vi "string to power value.vi"(9 "String":string) -> (10 "Power":T1)   [LabVIEW 2011]
uses:
  Power_config.ctl
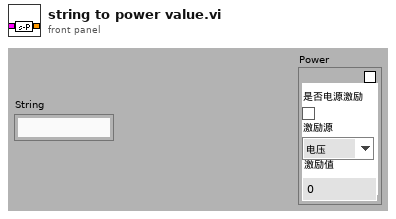
[diagram p1: front panel]
types:
  T1 = typedef "Power_config.ctl" = cluster{"power_en":bool, "Mode":enum16{"电压", "电流"}, "value":dbl, "Boolean":bool}
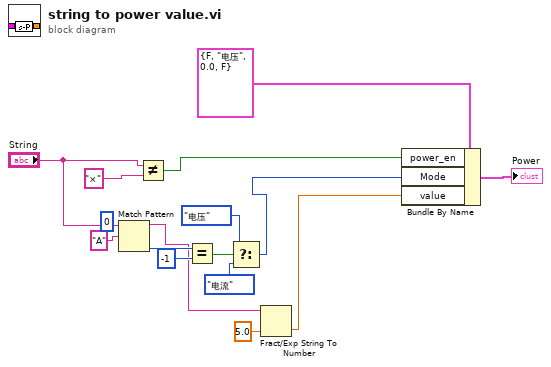
[diagram p0: block diagram]
diagram:
  (unwired) 0 ("offset past match")
  n1 = Match Pattern(string="String", regular expression="A") -> (before substring=w3:string, offset past match=w9:i32)  [unwired: 3 out]
  n2 = Not Equal?(x="String", y="×") -> (x != y?=w12:bool)
  n3 = Equal?(x=w9, y=-1) -> (x = y?=w7:bool)
  n4 = Select(t=enum16{"电压", "电流"}."电压" ("Mode"), s=w7, f=enum16{"电压", "电流"}."电流" ("Mode")) -> (s? t:f=w4:enum16{"电压", "电流"})
  n5 = Fract/Exp String To Number(string=w3, default (0 dbl)=5.0 ("default (0 DBL)")) -> (number=w2:dbl)  [unwired: 3 out]
  n6 = Bundle By Name(cluster=T1 {"power_en"=FALSE, "Mode"=enum."电压", "value"=0.0, "Boolean"=FALSE} ("Power"), "power_en"=w12, "Mode"=w4, "value"=w2) -> (→"Power":T1)
